vi "convert channels to lines.vi"(8 "error in (no error)":errorcluster, 11 "channels":refnum<class "TBM channel.lvclass">[](array[class])) -> (0 "error out":errorcluster, 3 "Lines":T1[](array[typedef]))   [LabVIEW 2013, in "Shared Memory configuration.lvclass"]
uses:
  Shared Memory configuration.lvclass
  Line.ctl
  <vilib>/NI/Tag Bus Module Framework/channel/TBM channel.lvclass
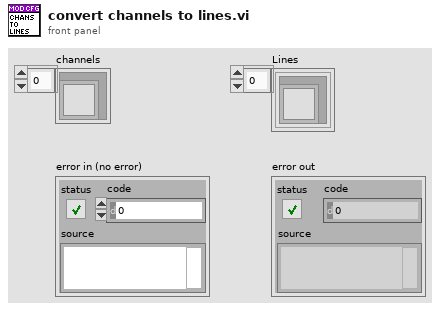
[diagram p1: front panel]
types:
  T1 = typedef "Shared Memory configuration.lvclass/Line.ctl" = cluster{"channel":refnum<class "TBM channel.lvclass">}
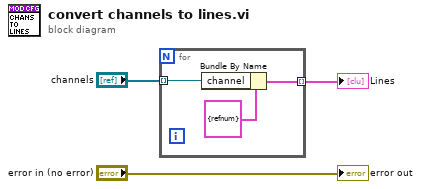
[diagram p0: block diagram]
diagram:
  n1 = for {
    tunnel: "channels" -> [w5] mode=indexing
    tunnel: [w4] -> w1 mode=indexing
    n2 = Bundle By Name(cluster=T1 {"channel"=refnum} ("Line"), "channel"=w5) -> (w4:T1)
  }
  "Lines" <- w1
  "error out" <- "error in (no error)"
